vi "solar_tcp Generate Error.vi"(10 "Source in":string) -> (2 "Source + Call Chain":string)   [LabVIEW 2018]
doc: "This adds the VI call chain to the Source string in."
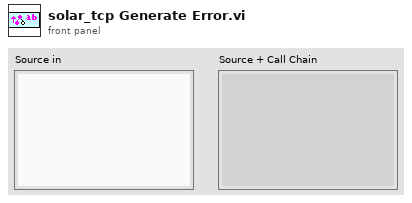
[diagram p1: front panel]
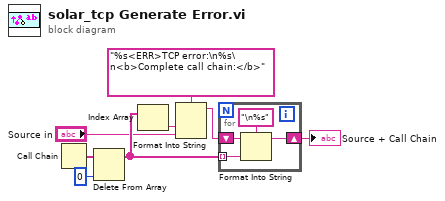
[diagram p0: block diagram]
diagram:
  n1 = Call Chain() -> (call chain=w5:string[])
  n2 = Delete From Array(array=w5, index=0) -> (array with subset deleted=w4:string[])  [unwired: 1 in, 1 out]
  n3 = Index Array(array=w4) -> (element=w7:string)  [unwired: 1 in]
  n4 = Format Into String(format string="%s<ERR>TCP error:\n%s\n<b>Complete call chain:</b>", w7, "Source in") -> (resulting string=w6:string)  [unwired: 2 in, 1 out]
  n5 = for {
    tunnel: w4 -> [w12] mode=indexing
    shift-right: [w11] -> w1
    shift-left: w6 -> [w10]
    n6 = Format Into String(format string="\n%s", initial string=w10, w12) -> (resulting string=w11:string)  [unwired: 1 in, 1 out]
  }
  "Source + Call Chain" <- w1
